vi "AddRoom.vi"(8 "error in (no error)":errorcluster, 10 "Room":refnum<class "Room.lvclass">, 11 "Maze in":refnum<class "Maze.lvclass">) -> (0 "error out":errorcluster, 3 "Maze out":refnum<class "Maze.lvclass">)   [LabVIEW 2020, in "Maze.lvclass"]
uses:
  Maze.lvclass
  ConcreteMazeSite/Room/Room.lvclass
  Maze.lvclass/Maze.ctl
  ConcreteMazeSite/Room/Room.lvclass/Room.ctl
  Private/Property/mRoomVec/Read mRoomVec.vi
  Private/Property/mRoomVec/Write mRoomVec.vi
  ConcreteMazeSite/Room/Property/roomNumber/Read roomNumber.vi
  MazeSite/MazeSite.lvclass
  Support/Class/ConsoleOutput.lvclass
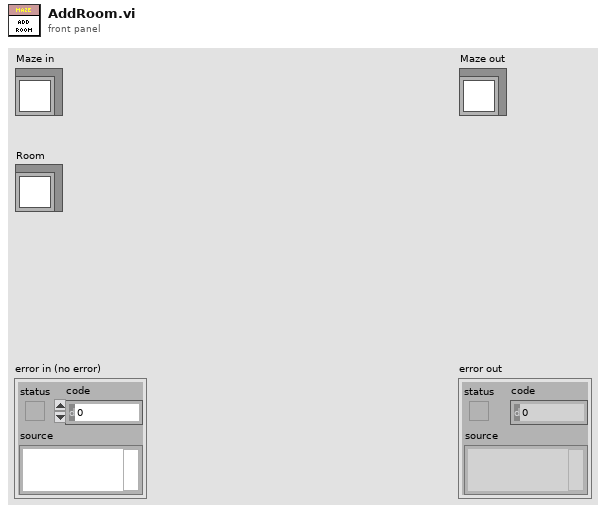
[diagram p1: front panel]
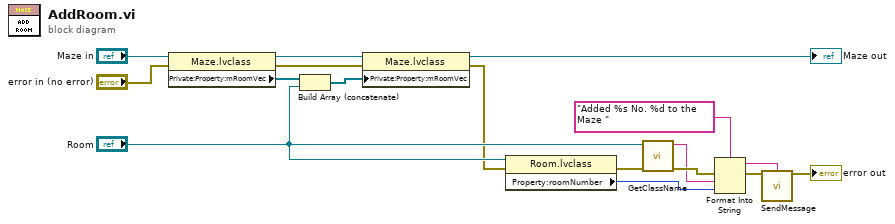
[diagram p0: block diagram]
diagram:
  n1 = property class="Maze.lvclass"(reference="Maze in", error in="error in (no error)") -> (reference out=w16:refnum<class "Maze.lvclass">, error out=w15:errorcluster, "Private:Property:mRoomVec"=w13:refnum<class "Room.lvclass">[])
  n2 = Build Array (concatenate)(w13, "Room") -> (w12:refnum<class "Room.lvclass">[])
  n3 = property class="Maze.lvclass"(reference=w16, error in=w15, "Private:Property:mRoomVec"=w12) -> (reference out=→"Maze out":refnum<class "Maze.lvclass">, error out=w5:errorcluster)
  n4 = property class="Room.lvclass"(reference="Room", error in=w5) -> (error out=w4:errorcluster, "Property:roomNumber"=w1:i32)  [unwired: 1 out]
  n5 = call "GetClassName.vi"("error in (no error)"=w4, "object"="Room") -> ("error out"=w3:errorcluster, "Class Name"=w2:string)  [unwired: 8 in]
  n6 = Format Into String(format string="Added %s No. %d to the Maze " ("Message"), error in=w3, w2, w1) -> (resulting string=w9:string, error out=w10:errorcluster)  [unwired: 1 in]
  n7 = call "SendMessage.vi"("Message"=w9, "error in (no error)"=w10) -> ("error out"=→"error out":errorcluster)  [unwired: 13 in]
